vi "Application Path.vi"() -> (1 "path":path)   [LabVIEW 2015]
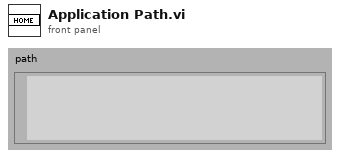
[diagram p1: front panel]
types:
  T1 = enum32{"invalid app kind", "Development System", "Run Time System", "Student Edition", "Embedded LabVIEW", "Evaluation", "Custom"}
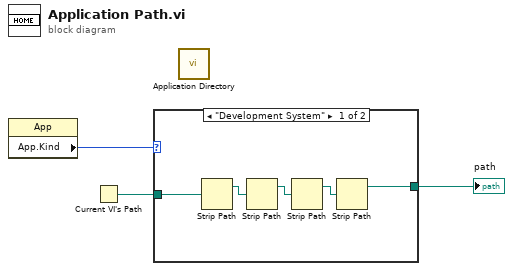
[diagram p0: block diagram]
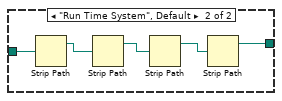
[diagram p2: hidden frame]
diagram:
  n1 = property class="App"() -> ("App.Kind"=w2:T1)  [unwired: 2 in, 2 out]
  n2 = Current VI's Path() -> (path=w3:path)
  n3 = case shown="\"Development System\"" w2 {
    tunnel: [w8 w9] -> w1
    tunnel: w3 -> [w4 w13]
    frame "Development System" {
      n4 = Strip Path(path=w4) -> (stripped path=w5:path)  [unwired: 1 out]
      n5 = Strip Path(path=w5) -> (stripped path=w6:path)  [unwired: 1 out]
      n6 = Strip Path(path=w6) -> (stripped path=w7:path)  [unwired: 1 out]
      n7 = Strip Path(path=w7) -> (stripped path=w8:path)  [unwired: 1 out]
    }
    frame "Run Time System", Default {
      n8 = Strip Path(path=w13) -> (stripped path=w12:path)  [unwired: 1 out]
      n9 = Strip Path(path=w12) -> (stripped path=w11:path)  [unwired: 1 out]
      n10 = Strip Path(path=w11) -> (stripped path=w10:path)  [unwired: 1 out]
      n11 = Strip Path(path=w10) -> (stripped path=w9:path)  [unwired: 1 out]
    }
  }
  "path" <- w1
  n12 = call <vilib>:"Application Directory.vi"() -> ()  [unwired: 1 out]
